vi "Kinect Global Status.vi"() -> ()   [LabVIEW 2011]
uses:
  <vilib>/vision/Image Controls.llb/IMAQ Image.ctl
  Microsoft.Kinect
panel:
  out "KinectSensor Ref":refnum<k24>
  out "DepthStream Callback Ref":refnum<k27>
  in  "DepthStream Ref":refnum<k24>
  in  "Frame ID":i32
  in  "Depth Image Queue":refnum<queue>
  in  "Kinect Status":T1={"Image Height"=0, "Image Width"=0, "Minimum Framerate"=0, "Maximum Framerate"=0, "Framerate"=25, "Near Mode"=TRUE, "Range"=0.0}
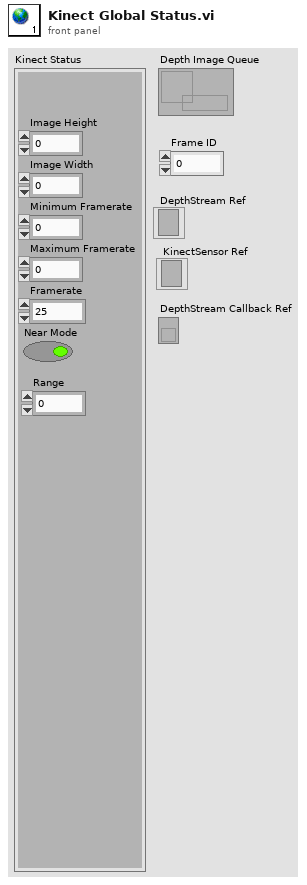
[diagram p1: front panel]
types:
  T1 = cluster{"Image Height":i32, "Image Width":i32, "Minimum Framerate":i32, "Maximum Framerate":i32, "Framerate":i32, "Near Mode":bool, "Range":sgl}
diagram:
